vi "Main_1.vi"() -> ()   [LabVIEW 2015]
panel:
  out "number (0 to 1)":dbl
  in  "Refresh":bool
  in  "Path":path
  in  "Numeric":dbl
  in  "Boolean":bool
  in  "stop":bool
  in  "OK":bool
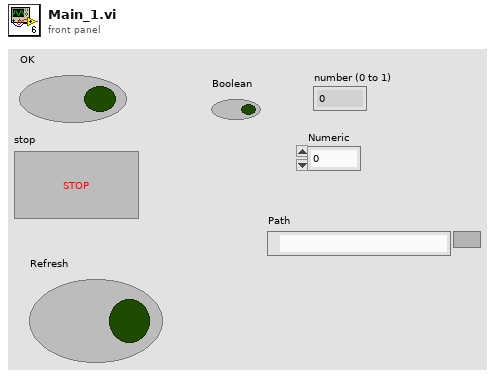
[diagram p1: front panel]
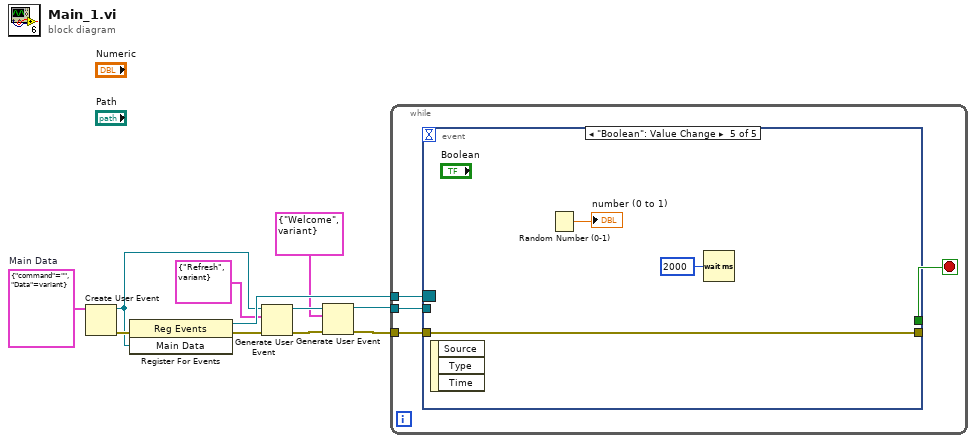
[diagram p0: block diagram]
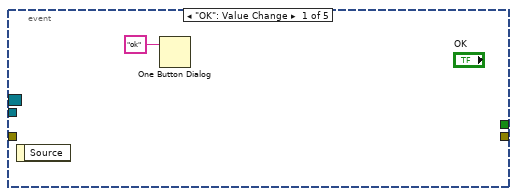
[diagram p2: hidden frame]
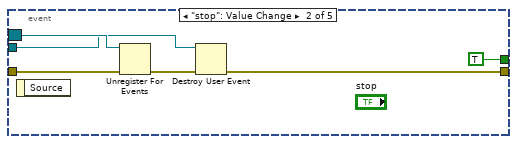
[diagram p3: hidden frame]
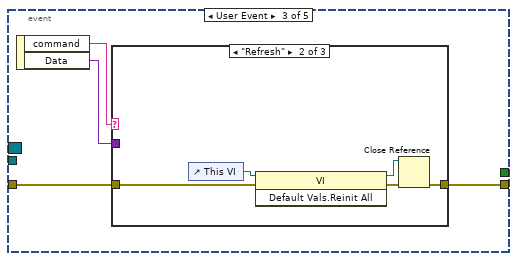
[diagram p4: hidden frame]
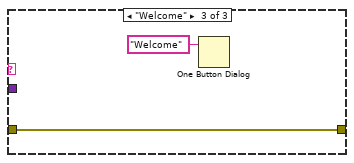
[diagram p6: hidden frame]
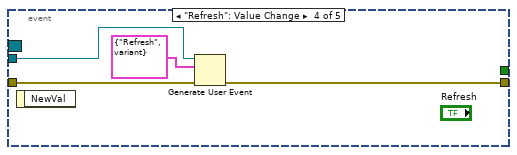
[diagram p7: hidden frame]
diagram:
  w11 = cluster{"command":string, "Data":variant} {"command"="", "Data"=variant}  # Main Data
  n1 = Create User Event(user event datatype=w11) -> (user event=w6:refnum<user-event>, error out=w8:errorcluster)  [unwired: 1 in]
  n2 = register-events(error in=w8, w6) -> (reference out=w10:refnum<event-registration>, error out=w7:errorcluster)  [unwired: 1 in]
  n3 = Generate User Event(user event=w6, event data cluster=cluster{"command":string, "Data":variant} {"command"="Refresh", "Data"=variant} ("event data"), error in=w7) -> (user event out=w3:refnum<user-event>, error out=w5:errorcluster)  [unwired: 1 in]
  n4 = Generate User Event(user event=w3, event data cluster=cluster{"command":string, "Data":variant} {"command"="Welcome", "Data"=variant} ("event data"), error in=w5) -> (user event out=w2:refnum<user-event>, error out=w4:errorcluster)  [unwired: 1 in]
  n5 = while {
    tunnel: w4 -> [w14]
    tunnel: w10 -> [w13]
    tunnel: w2 -> [w12]
    stop <- w15 stop-if-true
    n6 = event shown="[4] \"Boolean\": Value Change" {
      selector: w13 -> [_ w20 _ _ _]
      dyn-events: _ -> [_ _ _ _ _]
      timeout: _ -> [_ _ _ _ _]
      tunnel: [_ TRUE _ _ _] -> w15
      tunnel: w14 -> [_ w21 w24 w38 w40]
      tunnel: [_ w17 w23 w37 w40] -> _
      tunnel: w12 -> [_ w18 _ w35 _]
      event "OK": Value Change {
        n7 = event-data() -> ()  [unwired: 1 in, 1 out]
        n8 = One Button Dialog(message="ok") -> ()  [unwired: 1 in, 1 out]
      }
      event "stop": Value Change {
        n9 = event-data() -> ()  [unwired: 1 in, 1 out]
        n10 = Unregister For Events(event registration refnum=w20, error in=w21) -> (error out=w19:errorcluster)
        n11 = Destroy User Event(user event=w18, error in=w19) -> (error out=w17:errorcluster)
      }
      event User Event {
        n12 = event-data() -> ("command"=w26:string, "Data"=w25:variant)  [unwired: 1 in]
        n13 = case shown="\"Refresh\"" w26 {
          tunnel: w25 -> [_ _ _]
          tunnel: w24 -> [w27 w29 w33]
          tunnel: [w27 w28 w33] -> w23
          frame Default {
          }
          frame "Refresh" {
            n14 = control-ref of="This VI"() -> (w30:refnum<vi>)
            n15 = invoke class="VI" method="Default Vals.Reinit All"(reference=w30, error in=w29) -> (reference out=w32:refnum<vi>, error out=w31:errorcluster)  [unwired: 1 in, 1 out]
            n16 = Close Reference(reference=w32, error in (no error)=w31) -> (error out=w28:errorcluster)
          }
          frame "Welcome" {
            n17 = One Button Dialog(message="Welcome") -> ()  [unwired: 1 in, 1 out]
          }
        }
      }
      event "Refresh": Value Change {
        n18 = event-data() -> ()  [unwired: 1 in, 1 out]
        n19 = Generate User Event(user event=w35, event data cluster=cluster{"command":string, "Data":variant} {"command"="Refresh", "Data"=variant} ("event data"), error in=w38) -> (error out=w37:errorcluster)  [unwired: 1 in, 1 out]
      }
      event "Boolean": Value Change {
        n20 = event-data() -> ()  [unwired: 1 in, 3 out]
        n21 = Random Number (0-1)() -> (number: 0 to 1=→"number (0 to 1)":dbl)
        n22 = Wait (ms)(milliseconds to wait=u32 2000) -> ()  [unwired: 1 out]
      }
    }
  }
